vi "RobotDriveMecanumDrive_Cartesian_WithEncoder.vi"(0 "RobotDriveDevRef":T7={"DevStatus"={"status"=FALSE, "code"=0, "source"=""}, "Motors[]"=[], "Square Inputs"=FALSE, "Max Output"=1.0, "Isochronous"=FALSE}, 1 "Gyro Angle":dbl, 2 "RobotEncoderRef":T6, 5 "X":dbl, 9 "Y":dbl, 11 "error in (no error)":errorcluster, 12 "Rotation":dbl, 13 "Limit":dbl=1.0, 14 "PID gains":T1={"proportional gain (Kc)"=1.0, "integral time (Ti, min)"=0.01, "derivative time (Td, min)"=0.0} {"derivative time (Td, min)" format="%.3f"; "integral time (Ti, min)" format="%.3f"; "proportional gain (Kc)" format="%.3f"}) -> (4 "RobotDriveDevRef":T7={"DevStatus"={"status"=FALSE, "code"=0, "source"=""}, "Motors[]"=[], "Square Inputs"=FALSE, "Max Output"=1.0, "Isochronous"=FALSE}, 6 "Motor Values":dbl[](array[numeric]), 8 "Target Values":dbl[](array[numeric]), 15 "error out":errorcluster)   [LabVIEW 2013]
doc: "Configures the motors for holonomic driving. Holonomic driving allows you to move the robot in any direction without first rotating or maneuvering the robot.\n\nThis VI requires the robot to have either four omni-directional wheels and four motors mounted at 45 degree angles in the four corners of a square frame or to have four mecanum wheels driven by four motors.\n\nThe control input is intended to be connected directly to the X, Y, and Z axes of a joystick. The Y axis is inverted for you.\n\nThis software is licensed. Open the labview\\readme\\WPI Robotics Library Open Source License.txt file for more information."
uses:
  <vilib>/Rock Robotics/WPI/RobotDrive/WPI_RobotDriveDevRef.ctl
  <vilib>/Rock Robotics/WPI/MotorControl/WPI_MotorControlDeviceRef.ctl
  <vilib>/Rock Robotics/SystemInterfaces/Typedef/FPGA_TypedefDigitalModule.ctl
  <vilib>/Rock Robotics/SystemInterfaces/DIO/FPGA_DIOPWMChannel.ctl
  <vilib>/Rock Robotics/WPI/PWM/WPI_PWMDeadband.ctl
  <vilib>/Rock Robotics/WPI/CAN/Jaguar/SubVIs/WPI_CANJaguar_ControlMode.ctl
  <vilib>/Rock Robotics/WPI/PWM/WPI_PWMTransform_ConPane.ctl
  <vilib>/Rock Robotics/WPI/Encoder/WPI_EncoderDevRef.ctl
  <vilib>/Rock Robotics/SystemInterfaces/Encoder/FPGA_EncoderIdx.ctl
  <vilib>/Rock Robotics/SystemInterfaces/Counter/FPGA_CounterCtrSystemIndex.ctl
  <vilib>/Rock Robotics/WPI/Encoder/WPI_EncoderType.ctl
  <vilib>/Rock Robotics/SystemInterfaces/NetworkCommunication/NetComm_UsageReport_ResourceType.ctl
  <vilib>/Rock Robotics/WPI/RobotDrive/WPI_RobotDriveMotorSelectorEnum.ctl
  <vilib>/Rock Robotics/WPI/RobotDrive/WPI_RobotDriveSafetyCheck.vi
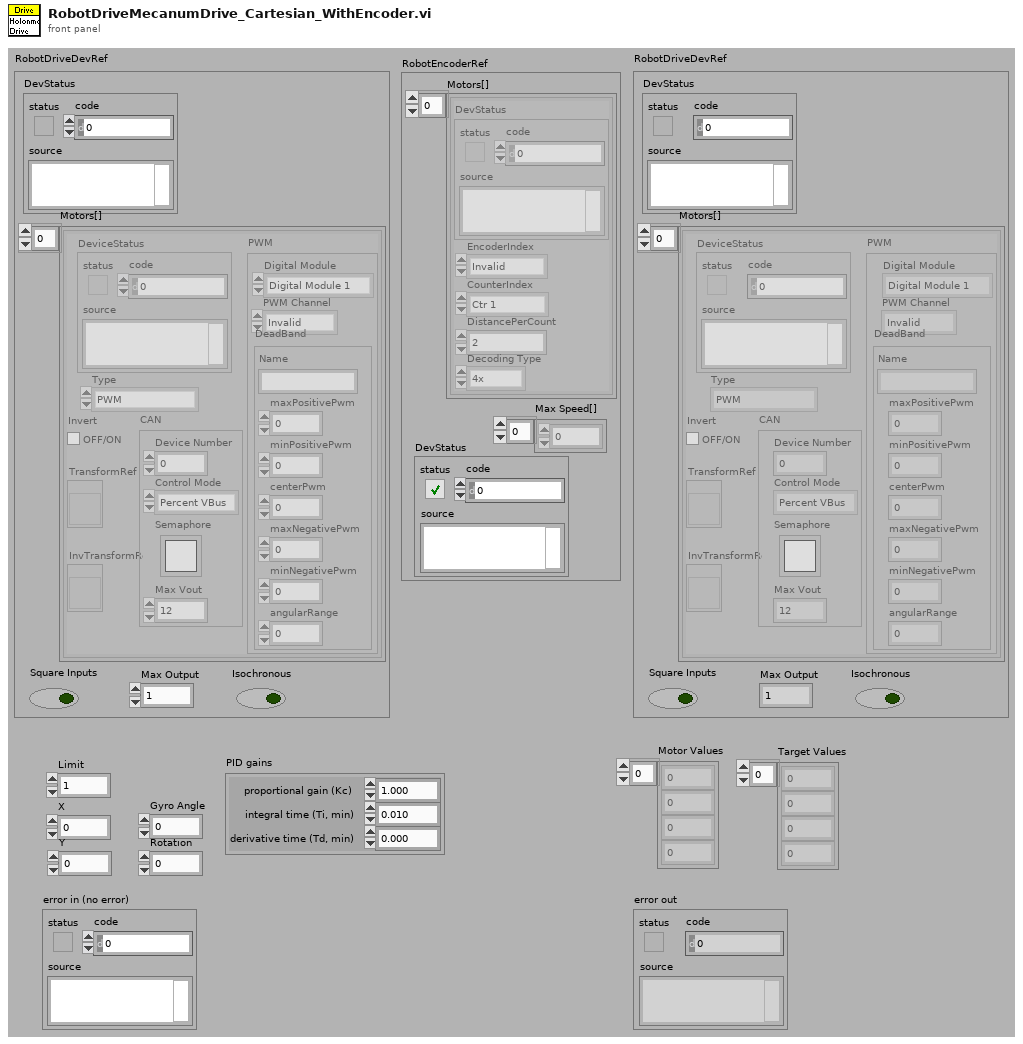
[diagram p1: front panel]
types:
  T1 = cluster{"proportional gain (Kc)":dbl, "integral time (Ti, min)":dbl, "derivative time (Td, min)":dbl}
  T2 = typedef "WPI_EncoderDevRef.ctl" = cluster{"DevStatus":errorcluster, "EncoderIndex":T3, "CounterIndex":T4, "DistancePerCount":dbl, "Decoding Type":T5}
  T3 = typedef "FPGA_EncoderIdx.ctl" = enum8{"Enc 0", "Enc 1", "Enc 2", "Enc 3", "Invalid"}
  T4 = typedef "FPGA_CounterCtrSystemIndex.ctl" = enum8{"Ctr 0", "Ctr 1", "Ctr 2", "Ctr 3", "Ctr 4", "Ctr 5", "Ctr 6", "Ctr 7", "Invalid"}
  T5 = typedef "WPI_EncoderType.ctl" = enum16{"1x", "2x", "4x"}
  T6 = cluster{"Motors[]":T2[], "DevStatus":errorcluster, "Max Speed[]":dbl[]}
  T7 = typedef "WPI_RobotDriveDevRef.ctl" = cluster{"DevStatus":errorcluster, "Motors[]":T8[], "Square Inputs":bool, "Max Output":dbl, "Isochronous":bool}
  T8 = typedef "WPI_MotorControlDeviceRef.ctl" = cluster{"DeviceStatus":errorcluster, "Type":enum16{"PWM", "CAN"}, "PWM":cluster{"Digital Module":T9, "PWM Channel":T10, "DeadBand":T11}, "CAN":cluster{"Device Number":u8, "Control Mode":T12, "Semaphore":T13, "Max Vout":dbl}, "Invert":bool, "TransformRef":T14, "InvTransformRef":T14}
  T9 = typedef "FPGA_TypedefDigitalModule.ctl" = enum16{"Digital Module 1", "Digital Module 2"}
  T10 = typedef "FPGA_DIOPWMChannel.ctl" = enum8{"PWM 1", "PWM 2", "PWM 3", "PWM 4", "PWM 5", "PWM 6", "PWM 7", "PWM 8", "PWM 9", "PWM 10", "Invalid"}
  T11 = typedef "WPI_PWMDeadband.ctl" = cluster{"Name":string, "maxPositivePwm":i32, "minPositivePwm":i32, "centerPwm":i32, "maxNegativePwm":i32, "minNegativePwm":i32, "angularRange":u16}
  T12 = typedef "WPI_CANJaguar_ControlMode.ctl" = enum8{"Percent VBus", "Current", "Speed", "Position", "Voltage"}
  T13 = typedef "Semaphore RefNum" = refnum<k1>
  T14 = typedef "WPI_PWMTransform_ConPane.ctl" = refnum<vi>
  T15 = typedef "NetComm_UsageReport_ResourceType.ctl" = enum8{"Controller", "Module", "Language", "CANPlugin", "Accelerometer", "ADXL345", "AnalogChannel", "AnalogTrigger", "AnalogTriggerOutput", "CANJaguar", "Compressor", "Counter", "Dashboard", "DigitalInput", "DigitalOutput", "DriverStationCIO", "DriverStationEIO", "DriverStationLCD", "Encoder", "GearTooth", "Gyro", "I2C", "Framework", "Jaguar", "Joystick", "Kinect", "KinectStick", "PIDController", "Preferences", "PWM", "Relay", "RobotDrive", "SerialPort", "Servo", "Solenoid", "SPI", "Task", "Ultrasonic", "Victor", "Button", "Command", "AxisCamera", "PCVideoServer", "SmartDashboard", "Talon", "HiTechnicColorSensor", "HiTechnicAccel", "HiTechnicCompass", "SRF08"}
  T16 = typedef "WPI_RobotDriveMotorSelectorEnum.ctl" = enum16{"Rear Left Motor", "Rear Right Motor", "Front Left Motor", "Front Right Motor"}
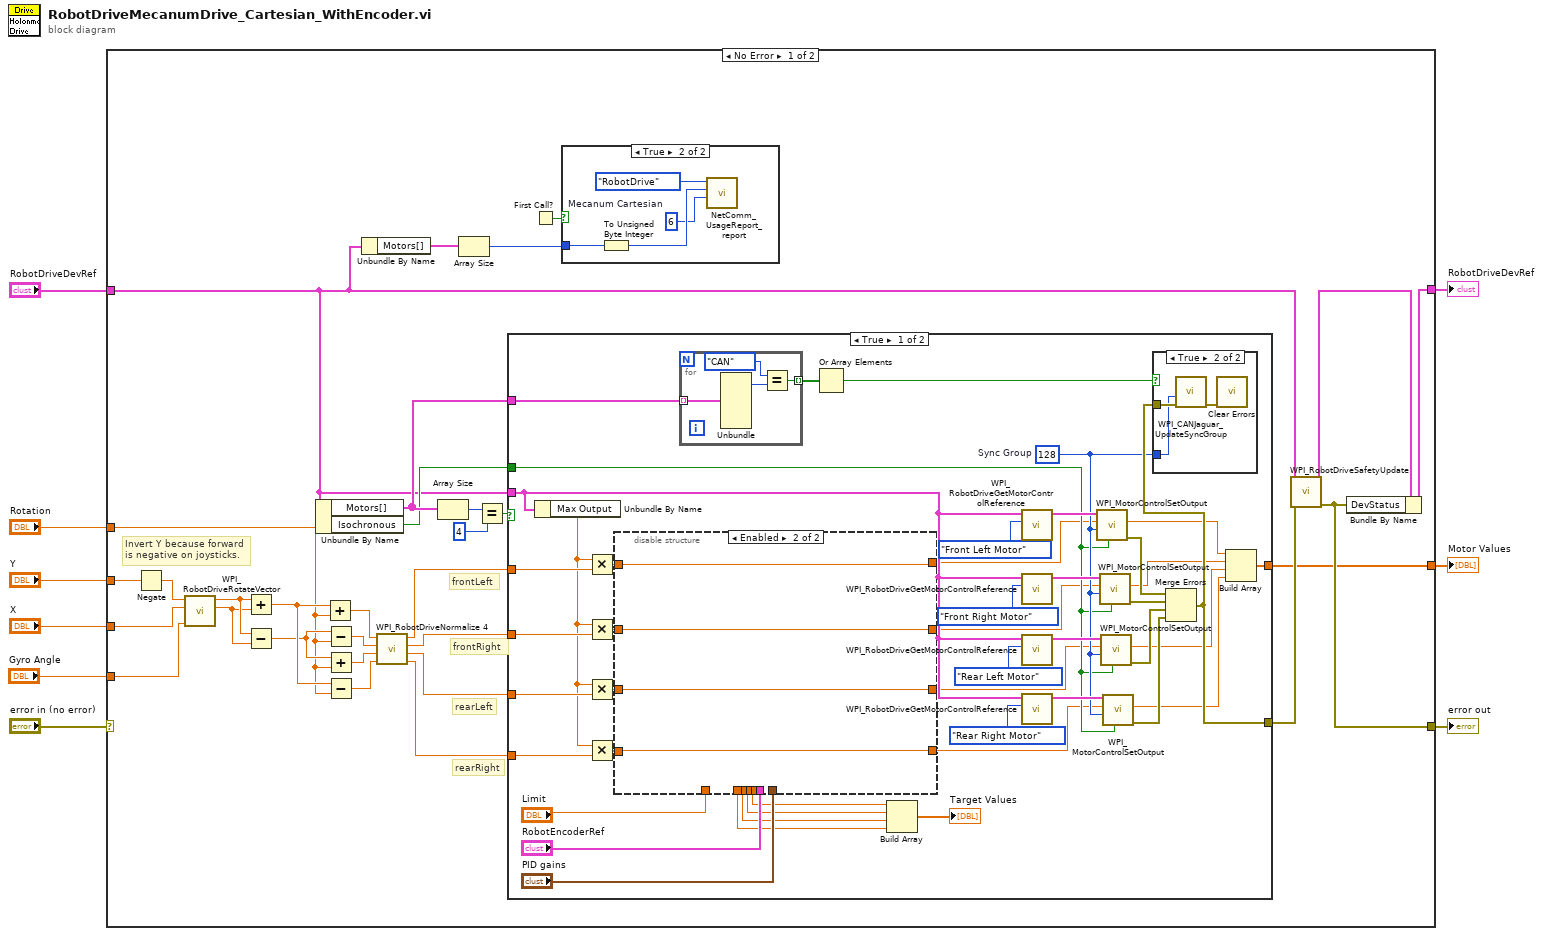
[diagram p0: block diagram]
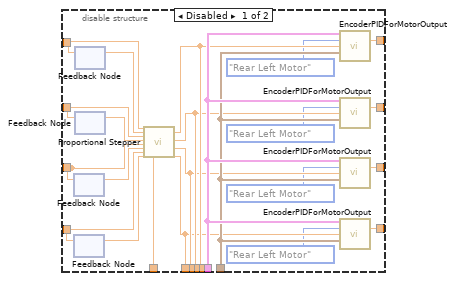
[diagram p3: hidden frame]
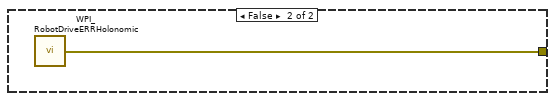
[diagram p5: hidden frame]
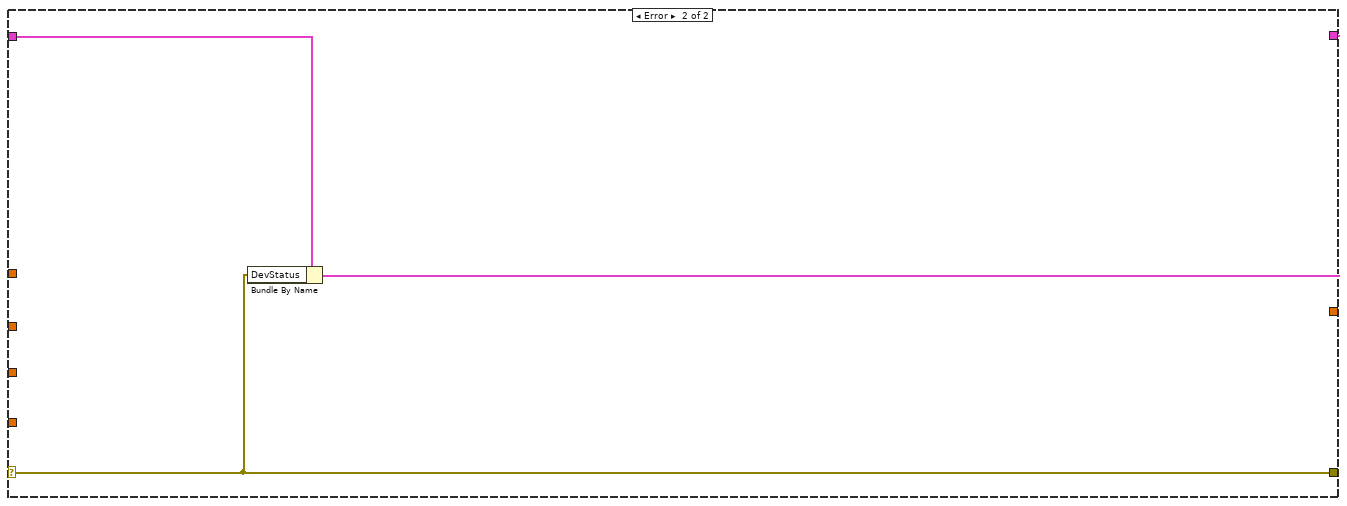
[diagram p6: hidden frame]
diagram:
  n1 = case shown="No Error" "error in (no error)" {
    selector: "error in (no error)" -> [_ w125]
    tunnel: "Y" -> [w22 _]
    tunnel: "X" -> [w27 _]
    tunnel: "RobotDriveDevRef" -> [w12 w127]
    tunnel: [w37 w126] -> w5
    tunnel: [w18 w125] -> w4
    tunnel: "Rotation" -> [w28 _]
    tunnel: "Gyro Angle" -> [w21 _]
    tunnel: [w11 _] -> w1
    frame No Error {
      # "Invert Y because forward is negative on joysticks."
      # "rearLeft"
      # "frontRight"
      # "rearRight"
      # "frontLeft"
      n2 = Negate(x=w22) -> (-x=w20:dbl)
      n3 = call <vilib>:"WPI_RobotDriveRotateVector.vi"("Angle"=w21, "X"=w27, "Y"=w20) -> ("X'"=w35:dbl, "Y'"=w36:dbl)  [unwired: 7 out]
      n4 = Add(x=w36, y=w35) -> (x+y=w33:dbl)
      n5 = Subtract(x=w36, y=w35) -> (x-y=w31:dbl)
      n6 = Unbundle By Name(w12) -> ("Motors[]"=w17:T8[], "Isochronous"=w16:bool)
      n7 = Add(x=w33, y=w28) -> (x+y=w29:dbl)
      n8 = Subtract(x=w31, y=w28) -> (x-y=w30:dbl)
      n9 = Add(x=w31, y=w28) -> (x+y=w32:dbl)
      n10 = Subtract(x=w33, y=w28) -> (x-y=w34:dbl)
      n11 = Unbundle By Name(w12) -> ("Motors[]"=w14:T8[])
      n12 = call <vilib>:"WPI_RobotDriveNormalize 4.vi"("D"=w34, "C"=w32, "B"=w30, "A"=w29) -> ("D'"=w24:dbl, "C'"=w23:dbl, "B'"=w25:dbl, "A'"=w26:dbl)
      n13 = Array Size(array=w17) -> (size(s)=w40:i32)
      n14 = Array Size(array=w14) -> (size(s)=w13:i32)
      n15 = Equal?(x=w40, y=4) -> (x = y?=w38:bool)
      n16 = case shown="True" w38 {
        tunnel: w26 -> [w89 _]
        tunnel: w25 -> [w88 _]
        tunnel: w12 -> [w77 _]
        tunnel: [w68 w124] -> w19
        tunnel: w23 -> [w83 _]
        tunnel: w24 -> [w82 _]
        tunnel: w17 -> [w69 _]
        tunnel: w16 -> [w66 _]
        tunnel: [w64 _] -> w11
        frame True {
          w67 = u8 128  # Sync Group
          n17 = Unbundle By Name(w77) -> ("Max Output"=w76:dbl)
          n18 = Multiply(x=w76, y=w89) -> (x*y=w60:dbl)
          n19 = Multiply(x=w76, y=w88) -> (x*y=w59:dbl)
          n20 = Multiply(x=w76, y=w83) -> (x*y=w58:dbl)
          n21 = Multiply(x=w76, y=w82) -> (x*y=w57:dbl)
          n22 = disable-structure shown="Enabled" {
            disable-tunnel: w60 -> [w112 w116]
            disable-tunnel: w59 -> [w111 w115]
            disable-tunnel: w58 -> [w110 w114]
            disable-tunnel: w57 -> [w109 w113]
            disable-tunnel: [w108 w113] -> w56
            disable-tunnel: [w107 w114] -> w55
            disable-tunnel: [w106 w115] -> w54
            disable-tunnel: [w105 w116] -> w53
            disable-tunnel: "Limit" -> [w104 _]
            disable-tunnel: "RobotEncoderRef" -> [w103 _]
            disable-tunnel: "PID gains" -> [w102 _]
            disable-tunnel: [w97 _] -> w48
            disable-tunnel: [w96 _] -> w47
            disable-tunnel: [w95 _] -> w46
            disable-tunnel: [w94 _] -> w45
            frame Disabled {
              n23 = feedback #1() -> (w100:dbl)  [unwired: 1 in]
              n24 = feedback-in #1(w110) -> ()
              n25 = feedback #2() -> (w99:dbl)  [unwired: 1 in]
              n26 = feedback-in #2(w109) -> ()
              n27 = feedback #3() -> (w101:dbl)  [unwired: 1 in]
              n28 = feedback-in #3(w112) -> ()
              n29 = feedback #4() -> (w98:dbl)  [unwired: 1 in]
              n30 = feedback-in #4(w111) -> ()
              n31 = call "Proportional Stepper.vi"("frontLeftNow"=w112, "frontLeftPrev"=w101, "frontRightNow"=w111, "frontRightPrev"=w98, "rearLeftNow"=w110, "rearLeftPrev"=w100, "rearRightNow"=w109, "rearRightPrev"=w99, "Limit"=w104) -> ("frontLeft'"=w97:dbl, "frontRight'"=w96:dbl, "rearLeft'"=w95:dbl, "rearRight'"=w94:dbl)  [unwired: 15 in]
              n32 = call "EncoderPIDForMotorOutput.vi"("RobotEncoderRef"=w103, "MotorIndex"=WPI_RobotDriveMotorSelectorEnum."Rear Left Motor", "Target"=w97, "PID gains"=w102) -> ("Output"=w105:dbl)  [unwired: 10 in, 1 out]
              n33 = call "EncoderPIDForMotorOutput.vi"("RobotEncoderRef"=w103, "MotorIndex"=WPI_RobotDriveMotorSelectorEnum."Rear Left Motor", "Target"=w96, "PID gains"=w102) -> ("Output"=w106:dbl)  [unwired: 10 in, 1 out]
              n34 = call "EncoderPIDForMotorOutput.vi"("RobotEncoderRef"=w103, "MotorIndex"=WPI_RobotDriveMotorSelectorEnum."Rear Left Motor", "Target"=w95, "PID gains"=w102) -> ("Output"=w107:dbl)  [unwired: 10 in, 1 out]
              n35 = call "EncoderPIDForMotorOutput.vi"("RobotEncoderRef"=w103, "MotorIndex"=WPI_RobotDriveMotorSelectorEnum."Rear Left Motor", "Target"=w94, "PID gains"=w102) -> ("Output"=w108:dbl)  [unwired: 10 in, 1 out]
            }
            frame Enabled {
            }
          }
          n36 = for {
            tunnel: w69 -> [w120] mode=indexing
            tunnel: [w117] -> w70 mode=indexing
            n37 = Unbundle(w120) -> ("Type"=w119:enum16{"PWM", "CAN"})  [unwired: 6 out]
            n38 = Equal?(x=enum16{"PWM", "CAN"}."CAN" ("Type"), y=w119) -> (x = y?=w117:bool)
          }
          n39 = Or Array Elements(Boolean array=w70) -> (logical OR=w71:bool)
          n40 = Build Array(w48, w47, w46, w45) -> (→"Target Values":dbl[])
          n41 = call <vilib>:"WPI_RobotDriveGetMotorControlReference.vi"("MotorIndex"=WPI_RobotDriveMotorSelectorEnum."Front Left Motor", "RobotDriveDevRef"=w77) -> ("MotorControlDeviceRef"=w87:T8)  [unwired: 9 out]
          n42 = call <vilib>:"WPI_RobotDriveGetMotorControlReference.vi"("MotorIndex"=WPI_RobotDriveMotorSelectorEnum."Front Right Motor", "RobotDriveDevRef"=w77) -> ("MotorControlDeviceRef"=w85:T8)  [unwired: 9 out]
          n43 = call <vilib>:"WPI_RobotDriveGetMotorControlReference.vi"("MotorIndex"=WPI_RobotDriveMotorSelectorEnum."Rear Left Motor", "RobotDriveDevRef"=w77) -> ("MotorControlDeviceRef"=w86:T8)  [unwired: 9 out]
          n44 = call <vilib>:"WPI_RobotDriveGetMotorControlReference.vi"("MotorIndex"=WPI_RobotDriveMotorSelectorEnum."Rear Right Motor", "RobotDriveDevRef"=w77) -> ("MotorControlDeviceRef"=w84:T8)  [unwired: 9 out]
          n45 = call <vilib>:"WPI_MotorControlSetOutput.vi"("Isochronous"=w66, "Sync Group"=w67, "Output"=w53, "MotorControlDevRef"=w87) -> ("error out"=w72:errorcluster, "Motor Output"=w65:dbl)  [unwired: 1 in, 5 out]
          n46 = call <vilib>:"WPI_MotorControlSetOutput.vi"("Isochronous"=w66, "Sync Group"=w67, "Output"=w54, "MotorControlDevRef"=w85) -> ("error out"=w73:errorcluster, "Motor Output"=w63:dbl)  [unwired: 1 in, 5 out]
          n47 = call <vilib>:"WPI_MotorControlSetOutput.vi"("Isochronous"=w66, "Sync Group"=w67, "Output"=w55, "MotorControlDevRef"=w86) -> ("error out"=w74:errorcluster, "Motor Output"=w62:dbl)  [unwired: 1 in, 5 out]
          n48 = call <vilib>:"WPI_MotorControlSetOutput.vi"("Isochronous"=w66, "Sync Group"=w67, "Output"=w56, "MotorControlDevRef"=w84) -> ("error out"=w75:errorcluster, "Motor Output"=w61:dbl)  [unwired: 1 in, 5 out]
          n49 = Merge Errors(w72, w73, w74, w75) -> (w68:errorcluster)
          n50 = case shown="True" w71 {
            tunnel: w68 -> [_ w122]
            tunnel: w67 -> [_ w121]
            frame False {
            }
            frame True {
              n51 = call <vilib>:"WPI_CANJaguar_UpdateSyncGroup.vi"("error in (no error)"=w122, "Sync Group"=w121) -> ("error out"=w123:errorcluster)  [unwired: 9 out]
              n52 = call <vilib>:"Clear Errors.vi"("error in (no error)"=w123) -> ()  [unwired: 7 out]
            }
          }
          n53 = Build Array(w65, w63, w62, w61) -> (w64:dbl[])
        }
        frame False {
          n54 = call <vilib>:"WPI_RobotDriveERRHolonomic.vi"() -> ("error out"=w124:errorcluster)
        }
      }
      n55 = First Call?() -> (First Call?: T/F=w15:bool)
      n56 = case shown="True" w15 {
        tunnel: w13 -> [_ w43]
        frame False {
        }
        frame True {
          w41 = u8 6  # Mecanum Cartesian
          n57 = To Unsigned Byte Integer(number=w43) -> (unsigned 8bit integer=w42:u8)
          n58 = call <vilib>:"NetComm_UsageReport_report.vi"("Context"=w41, "Instance Number"=w42, "Resource Type"=NetComm_UsageReport_ResourceType."RobotDrive") -> ()  [unwired: 9 in]
        }
      }
      n59 = call <vilib>:"WPI_RobotDriveSafetyUpdate.vi"("error in (no error)"=w19, "RobotDriveDevRef"=w12) -> ("error out"=w18:errorcluster, "RobotDriveDevRef"=w10:T7)  [unwired: 8 out]
      n60 = Bundle By Name(cluster=w10, "DevStatus"=w18) -> (w37:T7)
    }
    frame Error {
      n61 = Bundle By Name(cluster=w127, "DevStatus"=w125) -> (w126:T7)
    }
  }
  "error out" <- w4
  "RobotDriveDevRef" <- w5
  "Motor Values" <- w1
